vi "Read Profiles(for High-Speed Mode).vi"(8 "error in (no error)":errorcluster, 9 "Data Size (0: Auto Size)":u32, 10 "Read Req":T3={"Read Area"=TRUE, "Profile Pos"=0, "Read Profile No."=0, "Read Profile Cnt"=0, "Erase"=FALSE} {"Profile Pos" items=["CURRENT", "OLDEST", "SPECIFY"]}, 11 "Device ID (0)":i32) -> (0 "error out":errorcluster, 1 "Profile Rsp":T1, 2 "Profile Data":u32[](array[numeric]), 3 "Device ID out":i32, 5 "Profile Info":T2={"Profile Cnt"=1, "Envelope"=FALSE, " Profile Data Point"=0, " X Start"=0, " X Pitch"=0})   [LabVIEW 2014, in "Keyence LJ-V7000.lvlib"]
doc: "This function gets profile data.\nProfile data is stored in 0.01 ƒÊm units.\n\n<B>Note</B>:\nFor the details on the data stored in the profile data (storage order and size), see <B>10.3</B> in a manual of measuring instrument drivers."
uses:
  Keyence LJ-V7000.lvlib
  Clusters/Read Profile Req.ctl
  constant/Profile Pos.ctl
  Clusters/Profile Info.ctl
  Clusters/Read Profile Rsp.ctl
  constant/Driver VI No.ctl
  Private/vi/Low Level/Make DLL Param(Read Profile Req).vi
  Private/vi/Low Level/Make DLL Param(Read Profile Rsp).vi
  Private/vi/Low Level/Make VI Param(Read Profile Rsp).vi
panel:
  # "(c) 2012 KEYENCE CORPORATION.  ALL RIGHTS RESERVED."
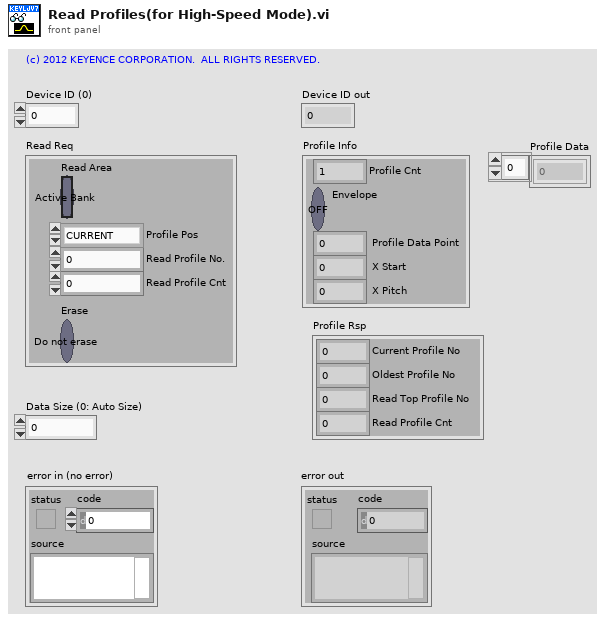
[diagram p1: front panel]
types:
  T1 = typedef "Keyence LJ-V7000.lvlib/Read Profile Rsp.ctl" = cluster{"Current Profile No":u32, "Oldest Profile No":u32, "Read Top Profile No":u32, "Read Profile Cnt":u8}
  T2 = typedef "Keyence LJ-V7000.lvlib/Profile Info.ctl" = cluster{"Profile Cnt":u8, "Envelope":bool, " Profile Data Point":u16, " X Start":i32, " X Pitch":i32}
  T3 = typedef "Keyence LJ-V7000.lvlib/Read Profile Req.ctl" = cluster{"Read Area":bool, "Profile Pos":T4, "Read Profile No.":u32, "Read Profile Cnt":u8, "Erase":bool}
  T4 = typedef "Keyence LJ-V7000.lvlib/Profile Pos.ctl" = u8
  T5 = typedef "Keyence LJ-V7000.lvlib/Driver VI No.ctl" = enum16{"Initialize", "Close", "Reboot Controller", "Return to Factory State", "Get System Error", "Clear System Error", "Trigger", "Start Batch Measurements", "Stop Batch Measurements", "Auto Zero", "Timing", "Reset", "Clear Memory", "Set Setting", "Get Setting", "Initialize Setting", "Reflect Setting", "Update Write Settings Area", "Check Status of Saving to Save Area", "Set Time", "Get Time", "Change Program", "Read Active Program Number", "Read Measurement Data", "Read Profiles(for High-Speed Mode)", "Read Batch Profiles(for High-Speed Mode)", "Read Profiles(for Advanced Mode)", "Read Batch Profiles(for Advanced Mode)", "Start Storage", "Stop Storage", "Read Storage Status", "Read Data Storage Data", "Read Profile Storage Data", "Read Batch Profile Storage Data", "Start High-Speed Data Communication", "Stop High-Speed Data Communication", "Read Profiles(for High-Speed Communication)"}
  T6 = cluster{"Profile Cnt":u8, u8, "reserve":u8, "reserve":u8, " Profile Data Point":u16, "reserve":u8, "reserve":u8, " X Start":i32, " XPitch":i32}
  T7 = cluster{"Current Profile No":u32, "Oldest Profile No":u32, "Read Top Profile No":u32, "Read Profile Cnt":u8, "reserve":u8, "reserve":u8, "reserve":u8}
  T8 = cluster{u8, "Profile Pos":T4, "reserve":u8, "reserve":u8, "Read Profile No.":u32, "Read Profile Cnt":u8, u8, "reserve":u8, "reserve":u8}
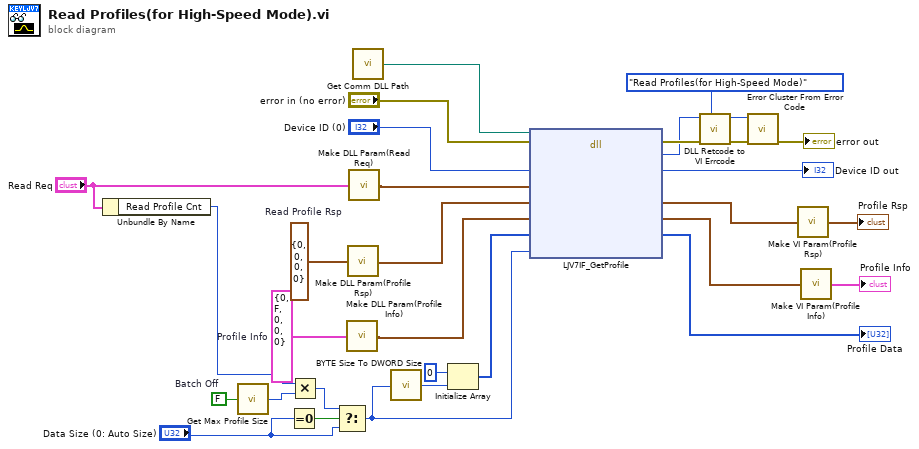
[diagram p0: block diagram]
diagram:
  w8 = FALSE  # Batch Off
  w25 = T2 {"Profile Cnt"=0, "Envelope"=FALSE, " Profile Data Point"=0, " X Start"=0, " X Pitch"=0}  # Profile Info
  w20 = T1 {"Current Profile No"=0, "Oldest Profile No"=0, "Read Top Profile No"=0, "Read Profile Cnt"=0}  # Read Profile Rsp
  n1 = Unbundle By Name("Read Req") -> ("Read Profile Cnt"=w1:u8)
  n2 = call "Get Max Profile Size.vi"("Batch On-Off"=w8) -> ("Profile Size"=w7:u32)  [unwired: 4 in]
  n3 = Equal To 0?(x="Data Size (0: Auto Size)") -> (x = 0?=w9:bool)
  n4 = Multiply(x=w1, y=w7) -> (x*y=w6:u32)
  n5 = Select(t=w6, s=w9, f="Data Size (0: Auto Size)") -> (s? t:f=w3:u32)
  n6 = call "Make DLL Param(Profile Info).vi"("Profile Info"=w25) -> ("DLL Parameter"=w26:T6)
  n7 = call-poly "Make DLL Param(Profile Rsp).vi"("Read Profile Rsp"=w20) -> ("pRsp"=w23:T7)
  n8 = call-poly "Make DLL Param(Read Req).vi"("Read Profile Req"="Read Req") -> ("pReq"=w24:T8)
  n9 = call "Get Comm DLL Path.vi"() -> ("Comm DLL Path"=w29:path)  [unwired: 1 in]
  n10 = call "BYTE Size To DWORD Size.vi"("BYTE Size"=w3) -> ("DWORD Size"=w10:u32)
  n11 = Initialize Array(u32 0, w10) -> (w4:u32[])
  n12 = dll-call lib="C:/Program Files/National Instruments/LabVIEW 2011/instr.lib/Keyence LJ-V7000/LJV7_IF.*" fn="LJV7IF_GetProfile"(path in=w29, error in="error in (no error)", "lDeviceId"="Device ID (0)", "pReq"=w24, "pRsp"=w23, "pProfileInfo"=w26, "pdwProfileData"=w4, "dwDataSize"=w3) -> (error out=w15:errorcluster, "lRetCode"=w14:i32, "lDeviceId"=→"Device ID out":i32, "pRsp"=w22:T7, "pProfileInfo"=w19:T6, "pdwProfileData"=→"Profile Data":u32[])  [unwired: 3 in, 1 out]
  n13 = call "DLL Retcode to VI Errcode.vi"("Driver VI No"=Driver_VI_No."Read Profiles(for High-Speed Mode)", "error in (no error)"=w15, "DLL Return Code"=w14) -> ("error out"=w17:errorcluster, "VI Error Code"=w16:i32)  [unwired: 7 in]
  n14 = call <vilib>:"Error Cluster From Error Code.vi"("error in (no error)"=w17, "error code (0)"=w16) -> ("error out"=→"error out":errorcluster)  [unwired: 7 in]
  n15 = call-poly "Make VI Param(Profile Rsp).vi"("pRsp"=w22) -> ("Read Profile Rsp"=→"Profile Rsp":T1)
  n16 = call "Make VI Param(Profile Info).vi"("pProfileInfo"=w19) -> ("Profile Info"=→"Profile Info":T2)
